vi "MGI RWA Read Strings from File.vi"(8 "Error In":errorcluster, 9 "Section Name":string, 11 "Path":path) -> (0 "Error Out":errorcluster, 1 "Found?":bool, 2 "String":string)   [LabVIEW 2016]
doc: "This VI was created for use with the Read/Write Anything VIs. It reads all the keys and their values from the specified section.\n\nAuthored by Robert C. Mortensen\nsupport@mooregoodideas.com\nwww.mooregoodideas.com\n\nCopyright (c) 2010, Moore Good Ideas, Inc.\n\nAll rights reserved.\n\nRedistribution and use in source and binary forms, with or without modification, are permitted provided that the following conditions are met:\n\n * Redistributions of source code must retain the above copyright notice, this list of conditions and the following disclaimer.\n * Redistributions in binary form must reproduce the above copyright notice, this list of conditions and the following disclaimer in the documentation and/or other materials provided with the distribution.\n * Neither the name of Moore Good Ideas, Inc. nor the names of its contributors may be used to endorse or promote products derived from this software without specific prior written permission.\n\nTHIS SOFTWARE IS PROVIDED BY THE COPYRIGHT HOLDERS AND CONTRIBUTORS \"AS IS\" AND ANY EXPRESS OR IMPLIED WARRANTIES, INCLUDING, BUT NOT LIMITED TO, THE IMPLIED WARRANTIES OF MERCHANTABILITY AND FITNESS FOR A PARTICULAR PURPOSE ARE DISCLAIMED. IN NO EVENT SHALL THE COPYRIGHT OWNER OR CONTRIBUTORS BE LIABLE FOR ANY DIRECT, INDIRECT, INCIDENTAL, SPECIAL, EXEMPLARY, OR CONSEQUENTIAL DAMAGES (INCLUDING, BUT NOT LIMITED TO, PROCUREMENT OF SUBSTITUTE GOODS OR SERVICES; LOSS OF USE, DATA, OR PROFITS; OR BUSINESS INTERRUPTION) HOWEVER CAUSED AND ON ANY THEORY OF LIABILITY, WHETHER IN CONTRACT, STRICT LIABILITY, OR TORT (INCLUDING NEGLIGENCE OR OTHERWISE) ARISING IN ANY WAY OUT OF THE USE OF THIS SOFTWARE, EVEN IF ADVISED OF THE POSSIBILITY OF SUCH DAMAGE."
uses:
  <userlib>/_MGI/Error Handling/MGI Suppress Error Code/MGI Suppress Error Code (Scalar).vi
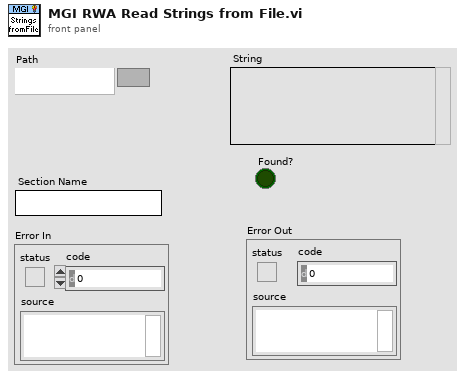
[diagram p1: front panel]
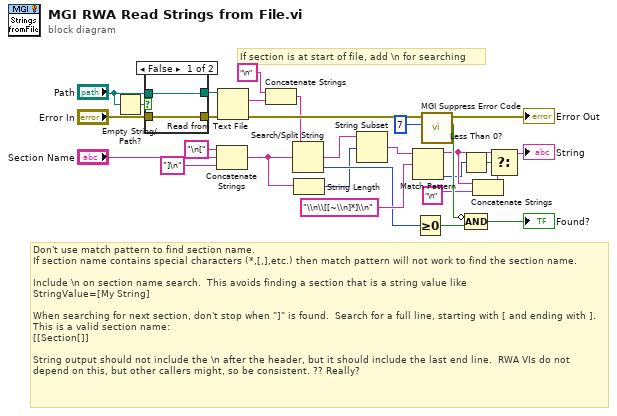
[diagram p0: block diagram]
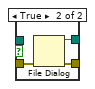
[diagram p2: hidden frame]
diagram:
  # "Don't use match pattern to find section name.\nIf section name contains special characters (*,[,],etc.) then match pattern will not work to find the section name.\n\nInclude \\n on section name search.  This avoids finding a section that is a string value like\nStringValue=[My String]\n\nWhen searching for next section, don't stop when \"]\" is found.  Search for a full line, starting with [ and ending with ].  This is a valid section name:\n[[Section[]]\n\nString output should not include the \\n after the header, but it should include the last end line.  RWA VIs do not depend on this, but other callers might, so be consistent. ?? Really?"
  # "If section is at start of file, add \\n for searching"
  n1 = Empty String/Path?(string/path="Path") -> (empty?=w21:bool)
  n2 = case shown="False" w21 {
    tunnel: "Error In" -> [w30 w34]
    tunnel: [w30 w33] -> w22
    tunnel: [w31 w32] -> w24
    tunnel: "Path" -> [w31 _]
    frame False {
    }
    frame True {
      n3 = File Dialog(8:w34) -> (0:w33:errorcluster, 3:w32:path)  [unwired: 8 out]
    }
  }
  n4 = Concatenate Strings("\n[" ("string"), "Section Name", "]\n" ("string")) -> (w8:string)
  n5 = Read from Text File(file (use dialog)=w24, error in=w22) -> (text=w13:string, error out=w18:errorcluster)  [unwired: 4 out]
  n6 = Concatenate Strings("\n" ("string"), w13) -> (w12:string)
  n7 = Search/Split String(string=w12, search string/char (-)=w8) -> (match + rest of string=w10:string, offset of match=w14:i32)  [unwired: 1 in, 1 out]
  n8 = String Length(string=w8) -> (length=w7:i32)
  n9 = String Subset(string=w10, offset (0)=w7) -> (substring=w9:string)  [unwired: 1 in]
  n10 = Match Pattern(string=w9, regular expression="\\n\\[[~\\n]*]\\n") -> (before substring=w4:string, offset past match=w2:i32)  [unwired: 3 out]
  n11 = Greater Or Equal To 0?(x=w14) -> (x >= 0?=w26:bool)
  n12 = call-poly <userlib>:"MGI Suppress Error Code.vi"("Error Code"=7, "Error In"=w18) -> ("Error Supressed?"=w15:bool, "Error Out"=→"Error Out":errorcluster)  [unwired: 4 in]
  n13 = Less Than 0?(x=w2) -> (x < 0?=w1:bool)
  n14 = Compound Arithmetic op=AND(invert w15, w26) -> (→"Found?":bool)
  n15 = Concatenate Strings(w4, "\n" ("string")) -> (w5:string)
  n16 = Select(t=w4, s=w1, f=w5) -> (s? t:f=→"String":string)
